vi "FullFile.vi"() -> ()   [LabVIEW 2012]
panel:
  in  "Full":cluster{"FullMIN":dbl, "FullMAX":dbl}={"FullMIN"=0.0, "FullMAX"=1.0}
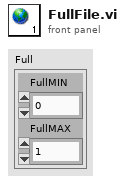
[diagram p1: front panel]
diagram:
